vi "4.vi"() -> ()   [LabVIEW 2015]
panel:
  out "XY图":cluster{dbl[], dbl[]}[](graph)
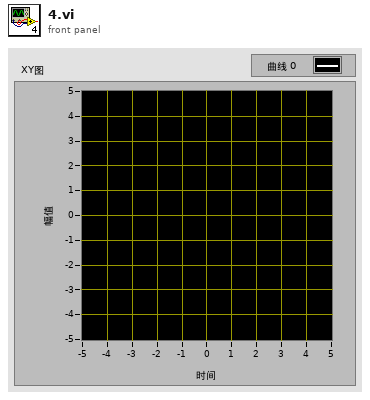
[diagram p1: front panel]
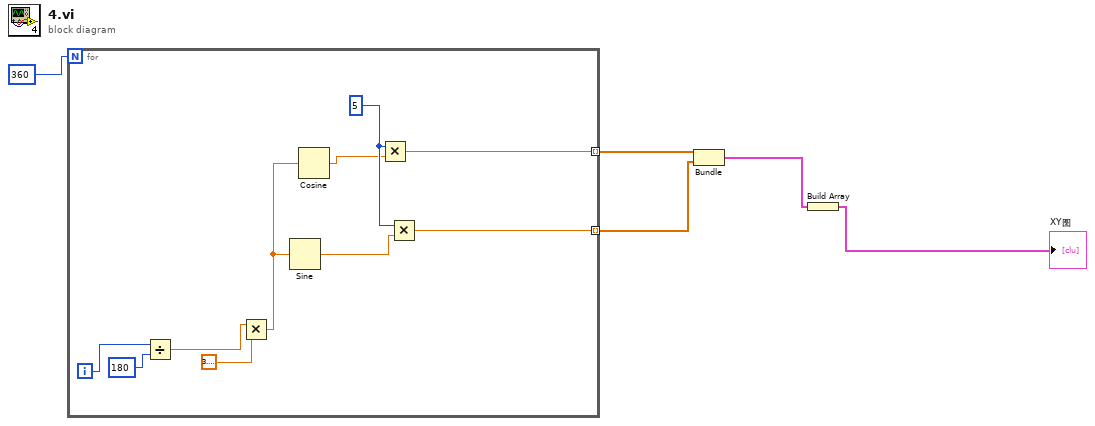
[diagram p0: block diagram]
diagram:
  n1 = for {
    N: 360 -> [_]
    tunnel: [w8] -> w4 mode=indexing
    tunnel: [w7] -> w3 mode=indexing
    i -> [w15]
    w10 = 5
    n2 = Divide(x=w15, y=180) -> (x/y=w13:dbl)
    n3 = Multiply(x=w13, y=3.141592653589793) -> (x*y=w11:dbl)
    n4 = Sine(x=w11) -> (sin(x)=w9:dbl)
    n5 = Cosine(x=w11) -> (cos(x)=w6:dbl)
    n6 = Multiply(x=w10, y=w6) -> (x*y=w8:dbl)
    n7 = Multiply(x=w10, y=w9) -> (x*y=w7:dbl)
  }
  n8 = Bundle(w4, w3) -> (w2:cluster{dbl[], dbl[]})  [unwired: 1 in]
  n9 = Build Array(w2) -> (→"XY图":cluster{dbl[], dbl[]}[])
